vi "resetAllChannels.vi"(8 "error in (no error)":errorcluster, 11 "BECHWCBasic in":refnum<class "BECHWCBasic.lvclass">) -> (0 "error out":errorcluster, 3 "BECHWCBasic out":refnum<class "BECHWCBasic.lvclass">)   [LabVIEW 2011, in "Hardware.lvlib" / "HWControllers.lvlib" / "BECHWCBasic.lvclass"]
uses:
  BECHWCBasic.lvclass
  BECHWCBasic.lvclass/BECHWCBasic.ctl
  Channels/VoltOutput/AnalogOutput.lvclass
  Channels/Digital/DigitalOutput.lvclass
  HWController.lvclass
  Tools/DatabaseHelpers/DbConnection/DeviceDataBase/deviceDataBase.lvclass
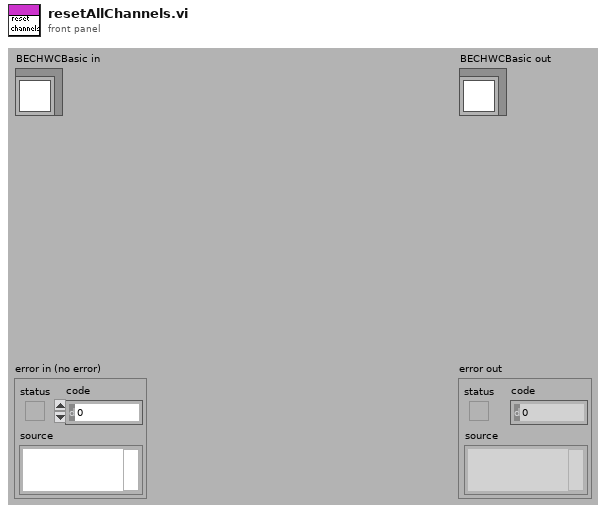
[diagram p1: front panel]
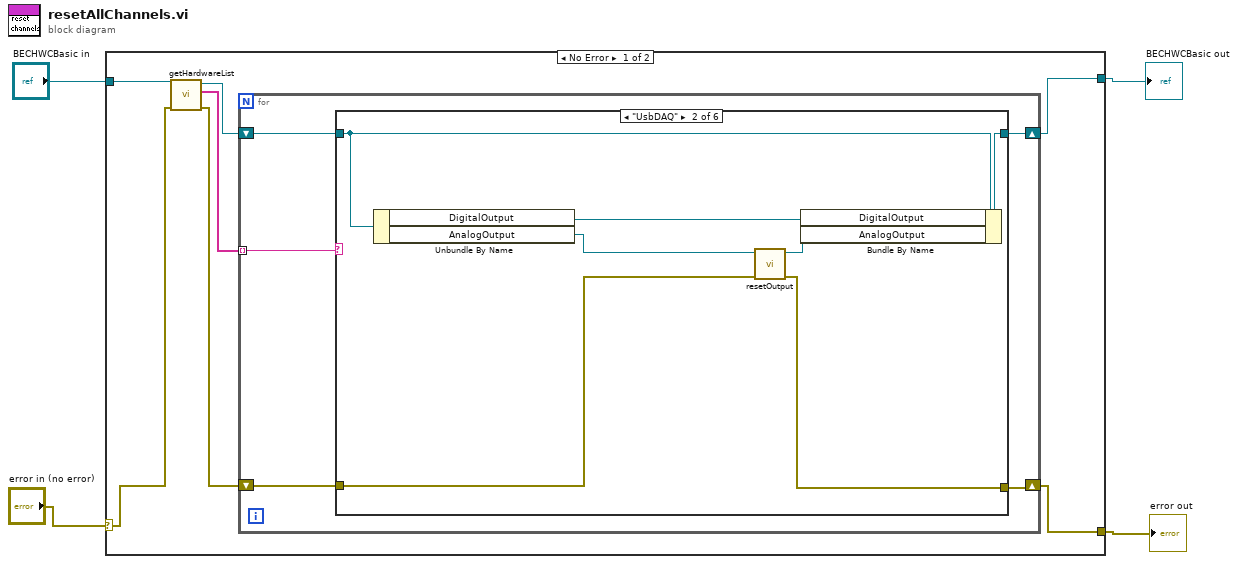
[diagram p0: block diagram]
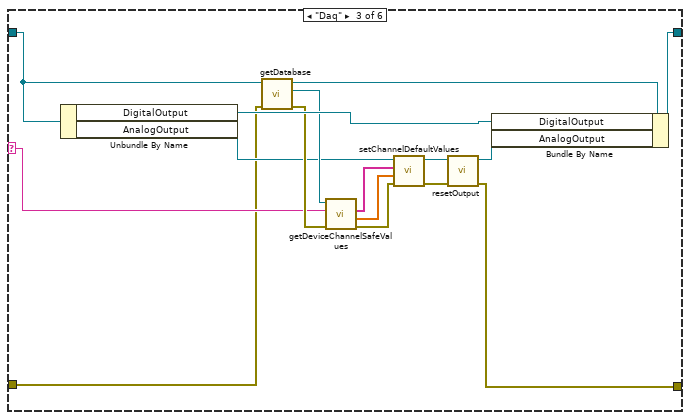
[diagram p3: hidden frame]
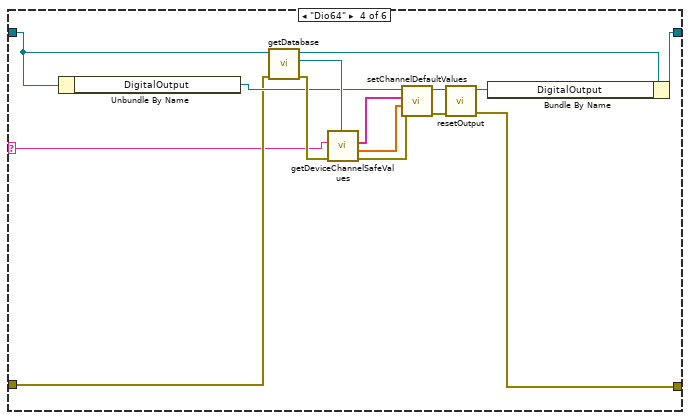
[diagram p4: hidden frame]
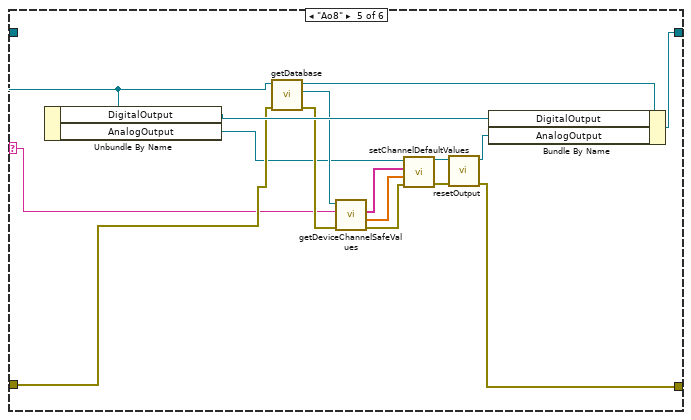
[diagram p5: hidden frame]
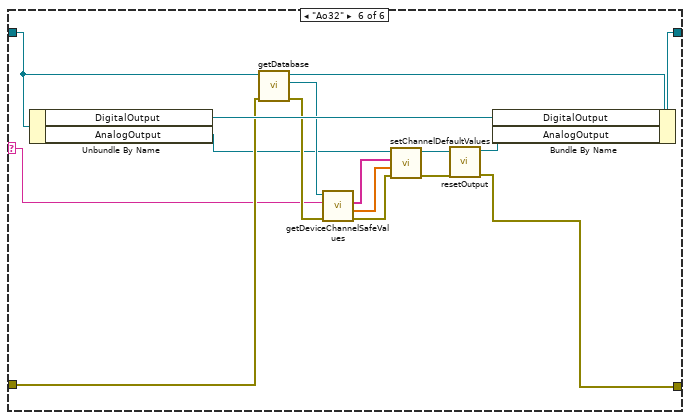
[diagram p6: hidden frame]
diagram:
  n1 = case shown="No Error" "error in (no error)" {
    selector: "error in (no error)" -> [w6 w89]
    tunnel: [w10 w89] -> w1
    tunnel: [w11 w90] -> w2
    tunnel: "BECHWCBasic in" -> [w9 w90]
    frame No Error {
      n2 = call "getHardwareList.vi"("error in (no error)"=w6, "HWController.lvclass in"=w9) -> ("error out"=w5:errorcluster, "HardwareList"=w8:string[], "HWController.lvclass out"=w7:refnum<class "BECHWCBasic.lvclass">)  [unwired: 7 in]
      n3 = for {
        tunnel: w8 -> [w13] mode=indexing
        shift-right: [w16] -> w11
        shift-left: w7 -> [w12]
        shift-right: [w14] -> w10
        shift-left: w5 -> [w15]
        n4 = case shown="\"UsbDAQ\"" w13 {
          selector: w13 -> [_ _ w28 w44 w59 w73]
          tunnel: w12 -> [w18 w25 w30 w48 w63 w79]
          tunnel: [w18 w24 w41 w56 w72 w88] -> w16
          tunnel: w15 -> [w17 w21 w26 w45 w61 w78]
          tunnel: [w17 w19 w38 w54 w69 w85] -> w14
          frame "No Hardware", Default {
          }
          frame "UsbDAQ" {
            n5 = Unbundle By Name(w25) -> ("DigitalOutput"=w20:refnum<class "DigitalOutput.lvclass">, "AnalogOutput"=w23:refnum<class "AnalogOutput.lvclass">)
            n6 = call-dynamic "resetOutput.vi"("error in (no error)"=w21, "AnalogOutput in"=w23) -> ("error out"=w19:errorcluster, "AnalogOutput out"=w22:refnum<class "AnalogOutput.lvclass">)  [unwired: 8 in]
            n7 = Bundle By Name(cluster=w25, "DigitalOutput"=w20, "AnalogOutput"=w22) -> (w24:refnum<class "BECHWCBasic.lvclass">)
          }
          frame "Daq" {
            n8 = Unbundle By Name(w30) -> ("DigitalOutput"=w39:refnum<class "DigitalOutput.lvclass">, "AnalogOutput"=w31:refnum<class "AnalogOutput.lvclass">)
            n9 = call "getDatabase.vi"("error in (no error)"=w26, "HWController in"=w30) -> ("error out"=w36:errorcluster, "deviceDataBase"=w37:refnum<class "deviceDataBase.lvclass">, "HWController out"=w29:refnum<class "BECHWCBasic.lvclass">)  [unwired: 7 in]
            n10 = call "getDeviceChannelSafeValues.vi"("error in (no error)"=w36, "device_name"=w28, "deviceDataBase in"=w37) -> ("error out"=w35:errorcluster, "SafeVaues"=w34:dbl[], "ChannelAddresses"=w33:string[])  [unwired: 5 in, 1 out]
            n11 = call "setChannelDefaultValues.vi"("error in (no error)"=w35, "calibratedValues"=w34, "channel_addresses"=w33, "AnalogOutput in"=w31) -> ("error out"=w27:errorcluster, "AnalogOutput out"=w32:refnum<class "AnalogOutput.lvclass">)  [unwired: 6 in]
            n12 = call-dynamic "resetOutput.vi"("error in (no error)"=w27, "AnalogOutput in"=w32) -> ("error out"=w38:errorcluster, "AnalogOutput out"=w40:refnum<class "AnalogOutput.lvclass">)  [unwired: 8 in]
            n13 = Bundle By Name(cluster=w29, "DigitalOutput"=w39, "AnalogOutput"=w40) -> (w41:refnum<class "BECHWCBasic.lvclass">)
          }
          frame "Dio64" {
            n14 = Unbundle By Name(w48) -> ("DigitalOutput"=w46:refnum<class "DigitalOutput.lvclass">)
            n15 = call "getDatabase.vi"("error in (no error)"=w45, "HWController in"=w48) -> ("error out"=w52:errorcluster, "deviceDataBase"=w53:refnum<class "deviceDataBase.lvclass">, "HWController out"=w47:refnum<class "BECHWCBasic.lvclass">)  [unwired: 7 in]
            n16 = call "getDeviceChannelSafeValues.vi"("error in (no error)"=w52, "device_name"=w44, "deviceDataBase in"=w53) -> ("error out"=w49:errorcluster, "SafeVaues"=w50:dbl[], "ChannelAddresses"=w51:string[])  [unwired: 5 in, 1 out]
            n17 = call-dynamic "setChannelDefaultValues.vi"("error in (no error)"=w49, "calibratedValues"=w50, "channel_addresses"=w51, "DigitalOutput in"=w46) -> ("error out"=w43:errorcluster, "DigitalOutput out"=w42:refnum<class "DigitalOutput.lvclass">)  [unwired: 6 in]
            n18 = call-dynamic "resetOutput.vi"("error in (no error)"=w43, "DigitalOutput in"=w42) -> ("error out"=w54:errorcluster, "DigitalOutput out"=w55:refnum<class "DigitalOutput.lvclass">)  [unwired: 8 in]
            n19 = Bundle By Name(cluster=w47, "DigitalOutput"=w55) -> (w56:refnum<class "BECHWCBasic.lvclass">)
          }
          frame "Ao8" {
            n20 = Unbundle By Name(w63) -> ("DigitalOutput"=w70:refnum<class "DigitalOutput.lvclass">, "AnalogOutput"=w60:refnum<class "AnalogOutput.lvclass">)
            n21 = call "getDatabase.vi"("error in (no error)"=w61, "HWController in"=w63) -> ("error out"=w67:errorcluster, "deviceDataBase"=w68:refnum<class "deviceDataBase.lvclass">, "HWController out"=w62:refnum<class "BECHWCBasic.lvclass">)  [unwired: 7 in]
            n22 = call "getDeviceChannelSafeValues.vi"("error in (no error)"=w67, "device_name"=w59, "deviceDataBase in"=w68) -> ("error out"=w66:errorcluster, "SafeVaues"=w65:dbl[], "ChannelAddresses"=w64:string[])  [unwired: 5 in, 1 out]
            n23 = call "setChannelDefaultValues.vi"("error in (no error)"=w66, "calibratedValues"=w65, "channel_addresses"=w64, "AnalogOutput in"=w60) -> ("error out"=w57:errorcluster, "AnalogOutput out"=w58:refnum<class "AnalogOutput.lvclass">)  [unwired: 6 in]
            n24 = call-dynamic "resetOutput.vi"("error in (no error)"=w57, "AnalogOutput in"=w58) -> ("error out"=w69:errorcluster, "AnalogOutput out"=w71:refnum<class "AnalogOutput.lvclass">)  [unwired: 8 in]
            n25 = Bundle By Name(cluster=w62, "DigitalOutput"=w70, "AnalogOutput"=w71) -> (w72:refnum<class "BECHWCBasic.lvclass">)
          }
          frame "Ao32" {
            n26 = Unbundle By Name(w79) -> ("DigitalOutput"=w86:refnum<class "DigitalOutput.lvclass">, "AnalogOutput"=w76:refnum<class "AnalogOutput.lvclass">)
            n27 = call "getDatabase.vi"("error in (no error)"=w78, "HWController in"=w79) -> ("error out"=w83:errorcluster, "deviceDataBase"=w84:refnum<class "deviceDataBase.lvclass">, "HWController out"=w75:refnum<class "BECHWCBasic.lvclass">)  [unwired: 7 in]
            n28 = call "getDeviceChannelSafeValues.vi"("error in (no error)"=w83, "device_name"=w73, "deviceDataBase in"=w84) -> ("error out"=w82:errorcluster, "SafeVaues"=w81:dbl[], "ChannelAddresses"=w80:string[])  [unwired: 5 in, 1 out]
            n29 = call "setChannelDefaultValues.vi"("error in (no error)"=w82, "calibratedValues"=w81, "channel_addresses"=w80, "AnalogOutput in"=w76) -> ("error out"=w77:errorcluster, "AnalogOutput out"=w74:refnum<class "AnalogOutput.lvclass">)  [unwired: 6 in]
            n30 = call-dynamic "resetOutput.vi"("error in (no error)"=w77, "AnalogOutput in"=w74) -> ("error out"=w85:errorcluster, "AnalogOutput out"=w87:refnum<class "AnalogOutput.lvclass">)  [unwired: 8 in]
            n31 = Bundle By Name(cluster=w75, "DigitalOutput"=w86, "AnalogOutput"=w87) -> (w88:refnum<class "BECHWCBasic.lvclass">)
          }
        }
      }
    }
    frame Error {
    }
  }
  "error out" <- w1
  "BECHWCBasic out" <- w2
